vi "get_Pump_state.vi"(8 "Error In":errorcluster, 10 "Насос in":T1={"Давление заданное"=0.3, "Давление MAX заданное"=100.0, "Давление в насосе"=0.0, "Давление в системе"=99.99, "Расход заданый"=0.0, "Расход текущий"=0.0, "Объём заданный"=0.0, "Объём текущий"=0.0, "Позиция насоса %"=0.0, "Ток двигателя"=0.0, "controlMsg"="", "Клапан k_sys"=FALSE, "Клапан k_res"=FALSE, "Клапан k_air"=FALSE, "Вверх"=FALSE, "Домой"=FALSE, "Вниз"=FALSE, "Старт расход"=FALSE, "Старт давление"=FALSE, "Сброс объёма"=FALSE, "Сброс давления Рсис"=FALSE, "Сброс давления Рнас"=FALSE, "Bits"={"plc_control"=FALSE, "lag_control"=FALSE, "mstop_control"=FALSE, "st_home"=FALSE, "error"=FALSE, "mstart"=FALSE, "pair"=FALSE, "startQ"=FALSE, "startP"=FALSE, "volume_Stop"=FALSE}} {"Ток двигателя" format="%#_5f"; "Расход текущий" format="%#_5f"; "Давление в системе" format="%.3f"; "Объём текущий" min=0.0 max=9999.0 step=0.0001 format="%#_5f"; "Объём заданный" min=0.0 max=9999.0 step=0.0001 format="%#_5f"; "Давление MAX заданное" min=0.0 max=100.0 step=0.01 format="%#_5f"; "Давление заданное" min=0.3 max=100.0 step=0.01 format="%#_5f"; "Расход заданый" min=0.0 max=40.0 step=0.0001 format="%#_5f"; "Давление в насосе" format="%.3f"; "Позиция насоса %" scale=0.0..100.0 scale format="%.2f"}, 11 "queue_Port in":refnum<queue>) -> (0 "Error Out":errorcluster, 3 "queue_Port out":refnum<queue>)   [LabVIEW 2023, in "pump_Lib.lvlib"]
uses:
  pump_Lib.lvlib
  TypeDef/pump_Type.ctl
panel:
  # "%"
  # "%"
  # "%"
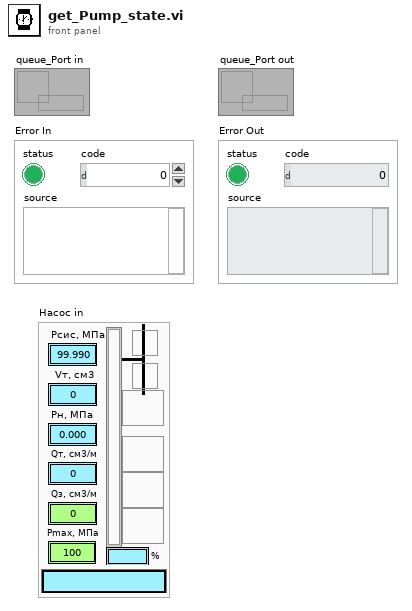
[diagram p1: front panel]
types:
  T1 = typedef "pump_Lib.lvlib/pump_Type.ctl" = cluster{"Давление заданное":dbl, "Давление MAX заданное":dbl, "Давление в насосе":dbl, "Давление в системе":dbl, "Расход заданый":dbl, "Расход текущий":dbl, "Объём заданный":dbl, "Объём текущий":dbl, "Позиция насоса %":dbl, "Ток двигателя":dbl, "controlMsg":string, "Клапан k_sys":bool, "Клапан k_res":bool, "Клапан k_air":bool, "Вверх":bool, "Домой":bool, "Вниз":bool, "Старт расход":bool, "Старт давление":bool, "Сброс объёма":bool, "Сброс давления Рсис":bool, "Сброс давления Рнас":bool, "Bits":cluster{"plc_control":bool, "lag_control":bool, "mstop_control":bool, "st_home":bool, "error":bool, "mstart":bool, "pair":bool, "startQ":bool, "startP":bool, "volume_Stop":bool}}
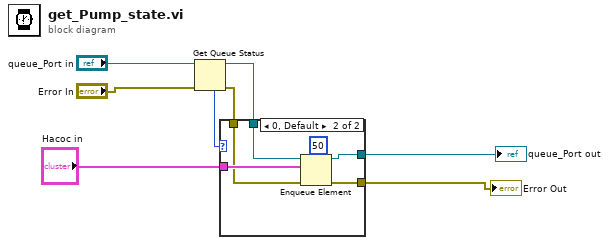
[diagram p0: block diagram]
diagram:
  n1 = Get Queue Status(queue="queue_Port in", error in (no error)="Error In") -> (queue out=w6:refnum<queue>, error out=w3:errorcluster, # elements in queue=w1:i32)  [unwired: 1 in, 5 out]
  n2 = case shown="0, Default" w1 {
    tunnel: w6 -> [w10 w15]
    tunnel: [w10 w14] -> w5
    tunnel: "Насос in" -> [_ w13]
    tunnel: w3 -> [w9 w12]
    tunnel: [w9 w11] -> w2
    frame 1 {
    }
    frame 0, Default {
      n3 = Enqueue Element(queue=w15, element=w13, timeout in ms (-1)=50, error in (no error)=w12) -> (queue out=w14:refnum<queue>, error out=w11:errorcluster)  [unwired: 1 out]
    }
  }
  "Error Out" <- w2
  "queue_Port out" <- w5
